vi "test Basic Launch.vi"(8 "error in (no error)":errorcluster, 11 "TestCase in":refnum<class "Monitor Test.lvclass">) -> (0 "error out":errorcluster, 3 "TestCase out":refnum<class "Monitor Test.lvclass">)   [LabVIEW 2017, in "Monitor Test.lvclass"]
uses:
  Monitor Test.lvclass
  monitored-actor-core/Source/Monitored Actor/Monitored Actor/Monitored Actor.lvclass
  C:/Program Files (x86)/National Instruments/LabVIEW 2017/vi.lib/ActorFramework/Actor/Actor.lvclass
  <vilib>/ActorFramework/Message Enqueuer/Message Enqueuer.lvclass/Message Enqueuer.ctl
  <vilib>/ActorFramework/Message Enqueuer/Enqueue.vi
  <vilib>/ActorFramework/Stop Msg/Stop Msg.lvclass
  C:/Program Files (x86)/National Instruments/LabVIEW 2017/vi.lib/ActorFramework/Message/Message.lvclass
  <vilib>/ActorFramework/Message Priority Queue/Priority Enqueue.vi
  <vilib>/ActorFramework/Actor/Actor.lvclass
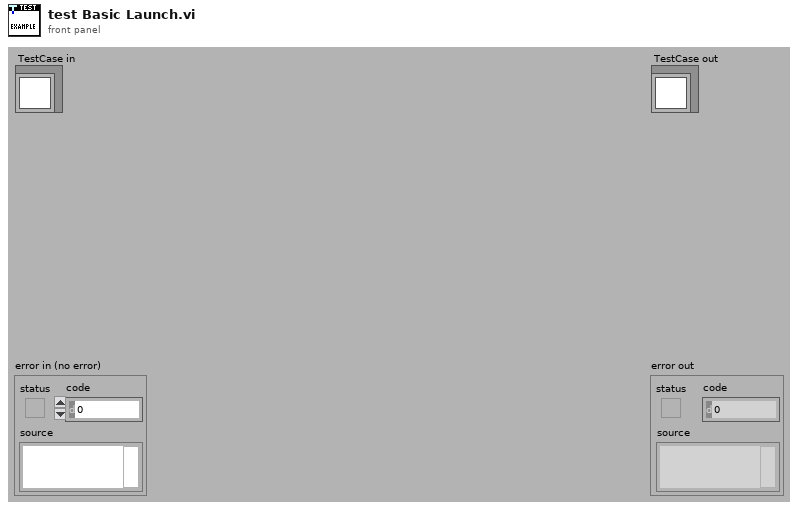
[diagram p1: front panel]
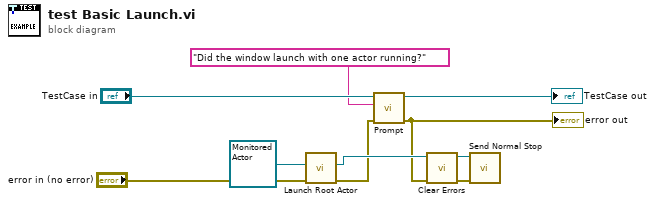
[diagram p0: block diagram]
diagram:
  n1 = call <vilib>:"Launch Root Actor.vi"("error in (no error)"="error in (no error)", "Actor"=refnum<class "Monitored Actor.lvclass"> refnum ("MGI-Monitored Actor Core.lvlib:Monitored Actor.lvclass")) -> ("error out"=w1:errorcluster, "Actor's Enqueuer"=w8:refnum<class "Message Enqueuer.lvclass">)  [unwired: 8 in]
  n2 = call "Prompt.vi"("error in (no error)"=w1, "Prompt"="Did the window launch with one actor running?", "Monitor Test in"="TestCase in") -> ("error out"=w3:errorcluster, "Monitor Test out"=→"TestCase out":refnum<class "Monitor Test.lvclass">)  [unwired: 7 in]
  "error out" <- w3
  n3 = call <vilib>:"Clear Errors.vi"("error in (no error)"=w3) -> ("error out"=w2:errorcluster)  [unwired: 5 in, 1 out]
  n4 = call <vilib>:"Send Normal Stop.vi"("error in (no error)"=w2, "Message Enqueuer"=w8) -> ()  [unwired: 9 in, 1 out]
